vi "Pre Launch Init.vi"(11 "CONTADOR_CON_LIMITES in":refnum<class "CONTADOR_CON_LIMITES.lvclass">) -> (0 "error out":errorcluster, 3 "CONTADOR_CON_LIMITES out":refnum<class "CONTADOR_CON_LIMITES.lvclass">)   [LabVIEW 2019, in "CONTADOR_CON_LIMITES.lvlib" / "CONTADOR_CON_LIMITES.lvclass"]
doc: "(<B>Filename</B>: Actor Framework.lvlib:Actor.lvclass:Pre Launch Init.vi)\n\nDefines behavior that occurs after the Launch Nested Actor method is invoked but before the actor's Actor Core method begins running.\n\nBy default, this method does nothing. A descendant class may override it to define behavior."
uses:
  CONTADOR_CON_LIMITES.lvclass
  CONTADOR_CON_LIMITES.lvclass/CONTADOR_CON_LIMITES.ctl
  <vilib>/ActorFramework/Actor/Actor.lvclass
panel:
  in  "LÍMITES":T1
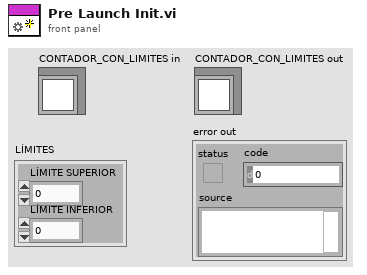
[diagram p1: front panel]
types:
  T1 = cluster{"LÍMITE SUPERIOR":dbl, "LÍMITE INFERIOR":dbl}
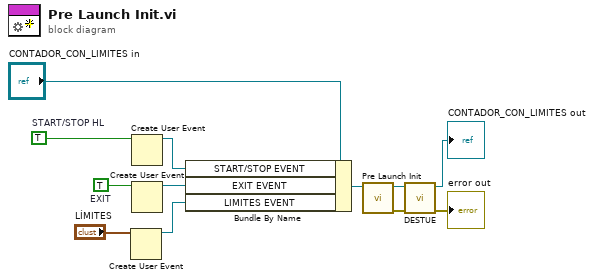
[diagram p0: block diagram]
diagram:
  w11 = TRUE  # EXIT
  w10 = TRUE  # START/STOP HL
  n1 = Create User Event(user event datatype="LÍMITES") -> (user event=w7:refnum<user-event>)  [unwired: 1 in, 1 out]
  n2 = Create User Event(user event datatype=w10) -> (user event=w5:refnum<user-event>)  [unwired: 1 in, 1 out]
  n3 = Create User Event(user event datatype=w11) -> (user event=w6:refnum<user-event>)  [unwired: 1 in, 1 out]
  n4 = Bundle By Name(cluster="CONTADOR_CON_LIMITES in", "START/STOP EVENT"=w5, "EXIT EVENT"=w6, "LIMITES EVENT"=w7) -> (w8:refnum<class "CONTADOR_CON_LIMITES.lvclass">)
  n5 = call-parent "Pre Launch Init.vi"("Actor in"=w8) -> ("error out"=w4:errorcluster, "Actor out"=w3:refnum<class "CONTADOR_CON_LIMITES.lvclass">)  [unwired: 9 in]
  n6 = call "DESTUE.vi"("error in (no error)"=w4, "CONTADOR_CON_LIMITES in"=w3) -> ("error out"=→"error out":errorcluster, "CONTADOR_CON_LIMITES out"=→"CONTADOR_CON_LIMITES out":refnum<class "CONTADOR_CON_LIMITES.lvclass">)  [unwired: 8 in]
